vi "TESTING ONLY.vi"() -> ()   [LabVIEW 2017]
uses:
  <vilib>/ActorFramework/LastAck/Last Ack.lvclass
  Configuration.lvclass
  C:/Program Files (x86)/National Instruments/LabVIEW 2017/vi.lib/ActorFramework/Actor/Actor.lvclass
  <vilib>/ActorFramework/Message Queue/Message Queue.lvclass/Message Queue.ctl
  <vilib>/ActorFramework/Message Dequeuer/Message Dequeuer.lvclass/Message Dequeuer.ctl
  <vilib>/ActorFramework/LastAck/Last Ack.lvclass/Last Ack.ctl
  <vilib>/ActorFramework/Message Priority Queue/Priority Dequeue.vi
  <vilib>/ActorFramework/Actor/Actor.lvclass
  <vilib>/ActorFramework/Message Queue/Message Queue.lvclass
  <vilib>/ActorFramework/Message Dequeuer/Message Dequeuer.lvclass
panel:
  in  "Configuration File Path":path=path "\\\\psf\\Home/Documents/Development/Networked Measurement System/Source/Framework/Measurements.ini"
  # "Run this test VI to launch the configuration dialog to act upon this file:"
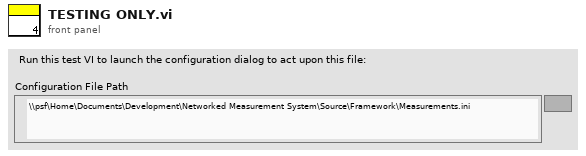
[diagram p1: front panel]
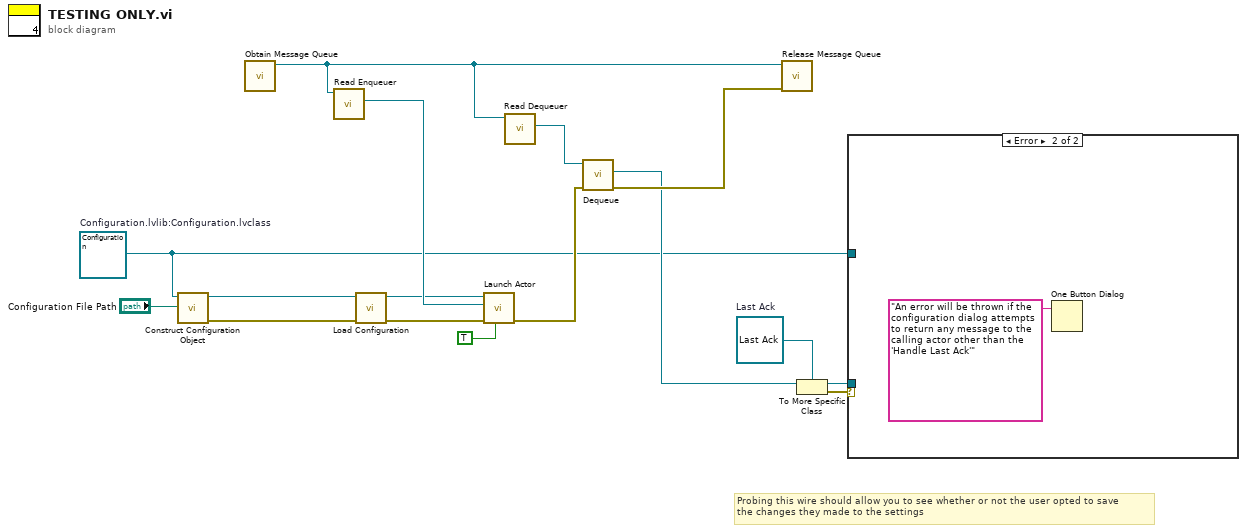
[diagram p0: block diagram]
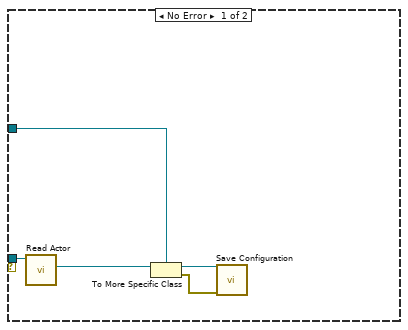
[diagram p2: hidden frame]
diagram:
  w2 = refnum<class "Configuration.lvclass"> refnum  # Configuration.lvlib:Configuration.lvclass
  w7 = refnum<class "Last Ack.lvclass"> refnum  # Last Ack
  # "Probing this wire should allow you to see whether or not the user opted to save\nthe changes they made to the settings"
  n1 = call "Construct Configuration Object.vi"("Configuration File Path"="Configuration File Path", "Configuration in"=w2) -> ("error out"=w4:errorcluster, "Configuration out"=w14:refnum<class "Configuration.lvclass">)  [unwired: 6 in, 2 out]
  n2 = call <vilib>:"Obtain Message Queue.vi"() -> ("Message Queue"=w12:refnum<class "Message Queue.lvclass">)  [unwired: 10 in, 1 out]
  n3 = call <vilib>:"Read Enqueuer.vi"("Message Queue"=w12) -> ("Message Enqueuer"=w16:refnum<class "Message Enqueuer.lvclass">)  [unwired: 10 in]
  n4 = call "Load Configuration.vi"("error in (no error)"=w4, "Configuration in"=w14) -> ("error out"=w3:errorcluster, "Configuration out"=w1:refnum<class "Configuration.lvclass">)  [unwired: 7 in, 1 out]
  n5 = call <vilib>:"Launch Actor.vi"("Open Actor Core front panel? (F)"=TRUE, "error in (no error)"=w3, "Actor-to-Caller Enqueuer"=w16, "Actor"=w1) -> ("error out"=w10:errorcluster)  [unwired: 6 in, 1 out]
  n6 = call <vilib>:"Read Dequeuer.vi"("Message Queue"=w12) -> ("Message Dequeuer"=w11:refnum<class "Message Dequeuer.lvclass">)  [unwired: 10 in]
  n7 = call <vilib>:"Dequeue.vi"("error in (no error)"=w10, "Message Dequeuer in"=w11) -> ("error out"=w9:errorcluster, "Message"=w8:refnum<class "Message.lvclass">)  [unwired: 5 in, 3 out]
  n8 = call <vilib>:"Release Message Queue.vi"("error in (no error)"=w9, "Message Queue"=w12) -> ()  [unwired: 8 in, 2 out]
  n9 = To More Specific Class(target class=w7, reference=w8) -> (specific class reference=w6:refnum<class "Last Ack.lvclass">, error out=w5:errorcluster)  [unwired: 1 in]
  n10 = case shown="Error" w5 {
    tunnel: w6 -> [w21 _]
    tunnel: w2 -> [w17 _]
    frame No Error {
      n11 = call <vilib>:"Read Actor.vi"("Last Ack"=w21) -> ("Actor"=w20:refnum<class "Actor.lvclass">)  [unwired: 10 in]
      n12 = To More Specific Class(target class=w17, reference=w20) -> (specific class reference=w19:refnum<class "Configuration.lvclass">, error out=w18:errorcluster)  [unwired: 1 in]
      n13 = call "Save Configuration.vi"("error in (no error)"=w18, "Configuration in"=w19) -> ()  [unwired: 7 in, 3 out]
    }
    frame Error {
      n14 = One Button Dialog(message="An error will be thrown if the configuration dialog attempts to return any message to the calling actor other than the 'Handle Last Ack'") -> ()  [unwired: 1 in, 1 out]
    }
  }
